vi "Write Cell Housekeeping.vi"(8 "error in":errorcluster, 10 "houseKeeping":T1, 11 "PAS Data in":refnum<class "PAS Data.lvclass">=refnum) -> (0 "error out":errorcluster, 3 "PAS Data out":refnum<class "PAS Data.lvclass">)   [LabVIEW 2014, in "PAS Data.lvclass"]
uses:
  PAS Data.lvclass
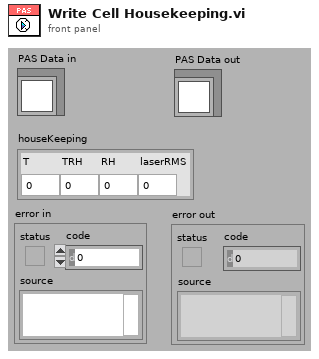
[diagram p1: front panel]
types:
  T1 = cluster{"T":sgl, "TRH":sgl, "RH":sgl, "laserRMS":sgl}
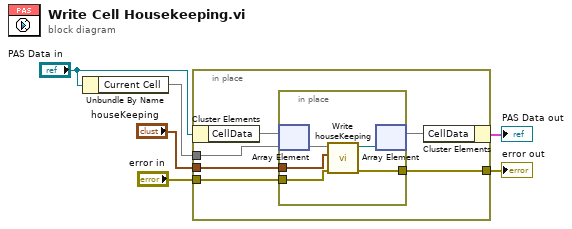
[diagram p0: block diagram]
diagram:
  n1 = Unbundle By Name("PAS Data in") -> ("Current Cell"=w4)
  n2 = in-place {
    in-place-border: w4 -> [w11]
    in-place-border: "houseKeeping" -> [w9]
    in-place-border: "error in" -> [w8]
    in-place-border: [w7] -> w1
    n3 = in-place-cluster #1("PAS Data in") -> ("CellData"=w12)
    n4 = in-place {
      in-place-border: w9 -> [w15]
      in-place-border: w8 -> [w14]
      in-place-border: [w13] -> w7
      n5 = in-place-array #2(w12, w11) -> (w17)
      n6 = call "Write houseKeeping.vi"("error in (no error)"=w14, "houseKeeping"=w15, "PAS Cell Data in"=w17) -> ("error out"=w13:errorcluster, "PAS Cell Data out"=w16:refnum<class "PAS Cell Data.lvclass">)  [unwired: 7 in]
      n7 = in-place-array #2(w16) -> (w10)  [unwired: 1 out]
    }
    n8 = in-place-cluster #1("CellData"=w10) -> (→"PAS Data out":cluster{})
  }
  "error out" <- w1
